vi "PathPlanner_GeomUtil_CoerceHeadingDegrees.vi"(11 "in Degrees":dbl) -> (3 "out Degrees":dbl)   [LabVIEW 2019, in "PathPlanner.lvlib"]
uses:
  PathPlanner.lvlib
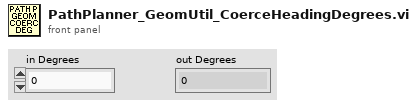
[diagram p1: front panel]
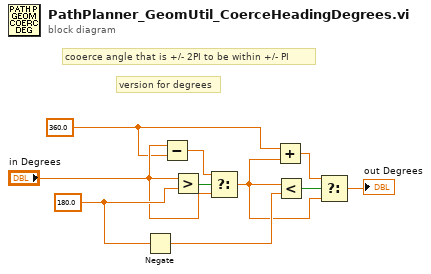
[diagram p0: block diagram]
diagram:
  w1 = 360.0
  w8 = 180.0
  # "version for degrees"
  # "cooerce angle that is +/- 2PI to be within +/- PI"
  n1 = Negate(x=w8) -> (-x=w7:dbl)
  n2 = Subtract(x="in Degrees", y=w1) -> (x-y=w9:dbl)
  n3 = Greater?(x="in Degrees", y=w8) -> (0:w10:bool)
  n4 = Select(t=w9, s=w10, f="in Degrees") -> (s? t:f=w5:dbl)
  n5 = Add(x=w1, y=w5) -> (x+y=w4:dbl)
  n6 = Less?(x=w5, y=w7) -> (x < y?=w6:bool)
  n7 = Select(t=w4, s=w6, f=w5) -> (s? t:f=→"out Degrees":dbl)
